vi "Send FC2 ILC Outputs.vi"(8 "error in (no error)":errorcluster, 11 "Model in":refnum<class "Model.lvclass">) -> (0 "error out":errorcluster, 3 "Model out":refnum<class "Model.lvclass">)   [LabVIEW 2015, in "Model.lvclass"]
uses:
  Model.lvclass
  Model.lvclass/Model.ctl
  <userlib>/Common/ILC/ILC/ILC.lvclass
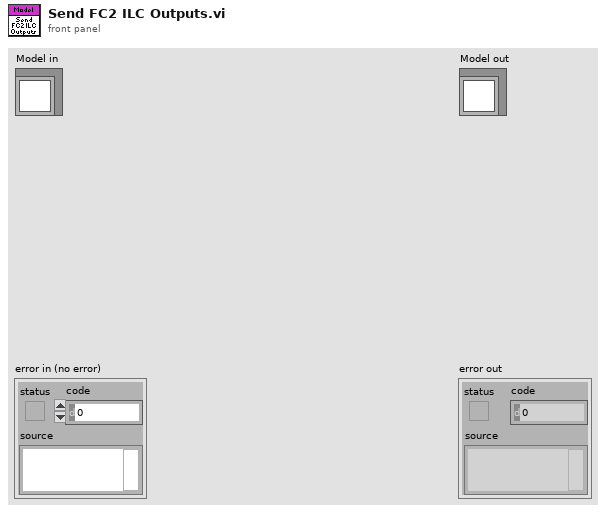
[diagram p1: front panel]
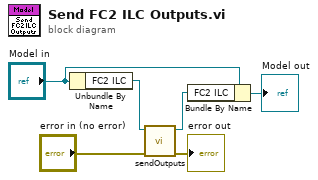
[diagram p0: block diagram]
diagram:
  n1 = Unbundle By Name("Model in") -> ("FC2 ILC"=w6:refnum<class "ILC.lvclass">)
  n2 = call <userlib>:"sendOutputs.vi"("error in (no error)"="error in (no error)", "ILC in"=w6) -> ("error out"=→"error out":errorcluster, "ILC out"=w3:refnum<class "ILC.lvclass">)  [unwired: 8 in]
  n3 = Bundle By Name(cluster="Model in", "FC2 ILC"=w3) -> (→"Model out":refnum<class "Model.lvclass">)
